vi "rad_BuildImageList.vi"(3 "error in":errorcluster, 4 "directory":bool, 5 "Image Path":path) -> (0 "error out":errorcluster, 2 "filenames":string[](array[string]))   [LabVIEW 2016]
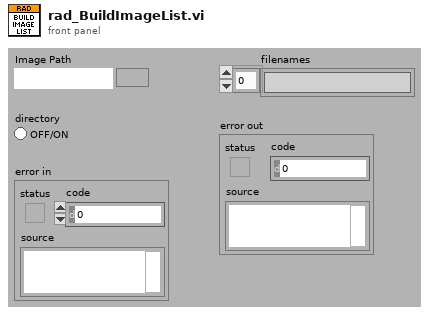
[diagram p1: front panel]
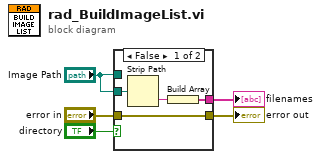
[diagram p0: block diagram]
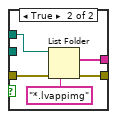
[diagram p2: hidden frame]
diagram:
  n1 = case shown="False" "directory" {
    tunnel: [w9 w13] -> w5
    tunnel: "Image Path" -> [_ w12]
    tunnel: "error in" -> [w8 w11]
    tunnel: [w8 w10] -> w3
    tunnel: "Image Path" -> [w7 _]
    frame False {
      n2 = Strip Path(path=w7) -> (name=w6:string)  [unwired: 1 out]
      n3 = Build Array(w6) -> (w9:string[])
    }
    frame True {
      n4 = List Folder(path=w12, pattern="*.lvappimg", error in=w11) -> (filenames=w13:string[], error out=w10:errorcluster)  [unwired: 1 in, 2 out]
    }
  }
  "filenames" <- w5
  "error out" <- w3
